vi "Get Pixels Below.vi"(9 "Pixel":T1={"Page"=0, "Row"=166, "Column"=84}, 11 "Pixmap Size":T1={"Page"=3, "Row"=200, "Column"=200}) -> (2 "Pixels Below":cluster{"Delta":dbl, "indices":T1}[](array[cluster]))   [LabVIEW 2018]
uses:
  Coords.ctl
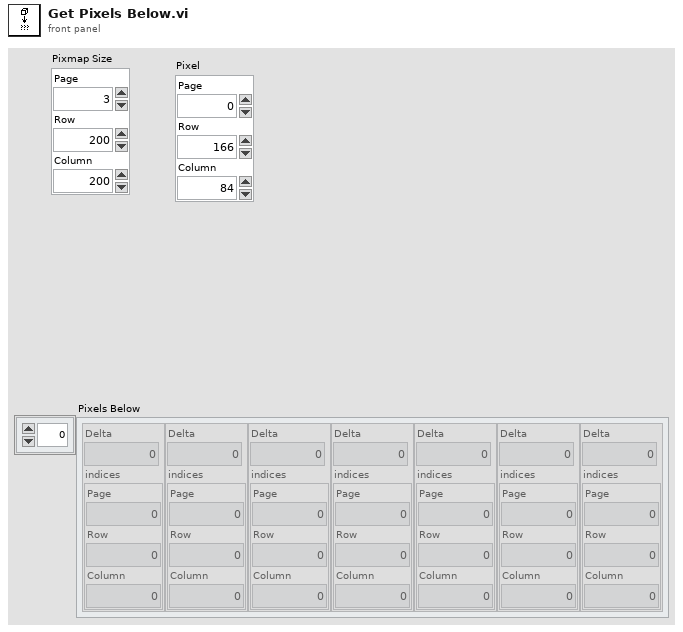
[diagram p1: front panel]
types:
  T1 = typedef "Coords.ctl" = cluster{"Page":i32, "Row":i32, "Column":i32}
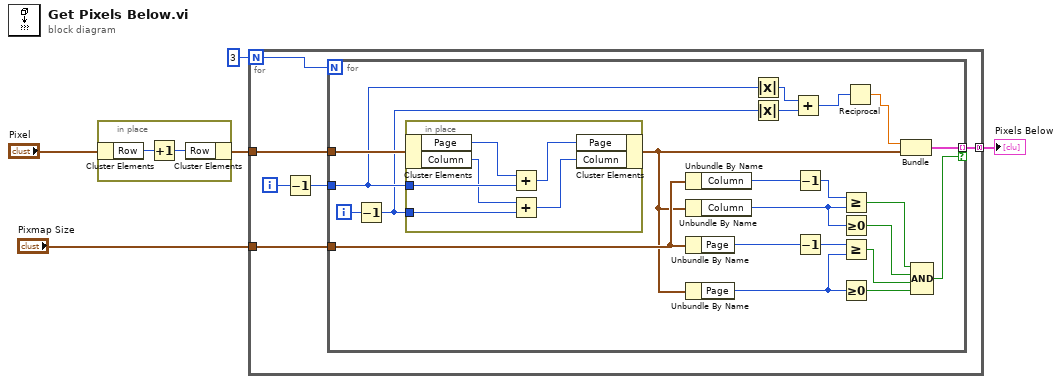
[diagram p0: block diagram]
diagram:
  n1 = in-place {
    n2 = in-place-cluster #1("Pixel") -> ("Row"=w7:i32)
    n3 = Increment(x=w7) -> (x+1=w6:i32)
    n4 = in-place-cluster #1("Row"=w6) -> (w4:T1)
  }
  n5 = for {
    N: 3 -> [w12]
    tunnel: w4 -> [w13]
    tunnel: "Pixmap Size" -> [w9]
    tunnel: [w8] -> w1 mode=concatenating
    i -> [w11]
    n6 = Decrement(x=w11) -> (x-1=w10:i32)
    n7 = for {
      N: w12 -> [_]
      tunnel: w13 -> [w34]
      tunnel: w10 -> [w21]
      tunnel: w9 -> [w30]
      tunnel: [w23] -> w8 mode=indexing if=w17
      i -> [w35]
      n8 = Decrement(x=w35) -> (x-1=w20:i32)
      n9 = in-place {
        in-place-border: w21 -> [w40]
        in-place-border: w20 -> [w36]
        n10 = in-place-cluster #2(w34) -> ("Page"=w41:i32, "Column"=w38:i32)
        n11 = Add(x=w41, y=w40) -> (x+y=w39:i32)
        n12 = Add(x=w38, y=w36) -> (x+y=w37:i32)
        n13 = in-place-cluster #2("Page"=w39, "Column"=w37) -> (w18:T1)
      }
      n14 = Unbundle By Name(w30) -> ("Column"=w32:i32)
      n15 = Unbundle By Name(w18) -> ("Column"=w33:i32)
      n16 = Unbundle By Name(w30) -> ("Page"=w25:i32)
      n17 = Unbundle By Name(w18) -> ("Page"=w14:i32)
      n18 = Absolute Value(x=w21) -> (abs(x)=w22:i32)
      n19 = Absolute Value(x=w20) -> (abs(x)=w19:i32)
      n20 = Add(x=w22, y=w19) -> (x+y=w16:i32)
      n21 = Decrement(x=w32) -> (x-1=w31:i32)
      n22 = Decrement(x=w25) -> (x-1=w24:i32)
      n23 = Greater Or Equal?(x=w31, y=w33) -> (x >= y?=w29:bool)
      n24 = Greater Or Equal To 0?(x=w33) -> (x >= 0?=w28:bool)
      n25 = Greater Or Equal?(x=w24, y=w14) -> (x >= y?=w27:bool)
      n26 = Greater Or Equal To 0?(x=w14) -> (x >= 0?=w26:bool)
      n27 = Reciprocal(x=w16) -> (1/x=w15:dbl)
      n28 = Bundle(w15, "Pixel"=w18) -> (w23:cluster{dbl, "Pixel":T1})  [unwired: 1 in]
      n29 = Compound Arithmetic op=AND(w29, w28, w27, w26) -> (w17:bool)
    }
  }
  "Pixels Below" <- w1
